vi "for_loop-2d.vi"() -> ()   [LabVIEW 2012]
panel:
  out "column  iterations":i32
  out "Rows":i32
  out "Array":i32[][](array[numeric])
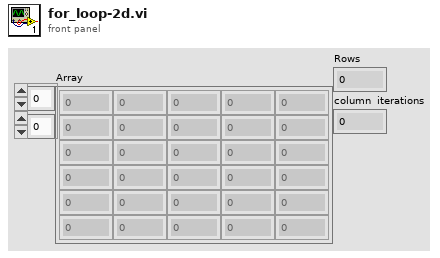
[diagram p1: front panel]
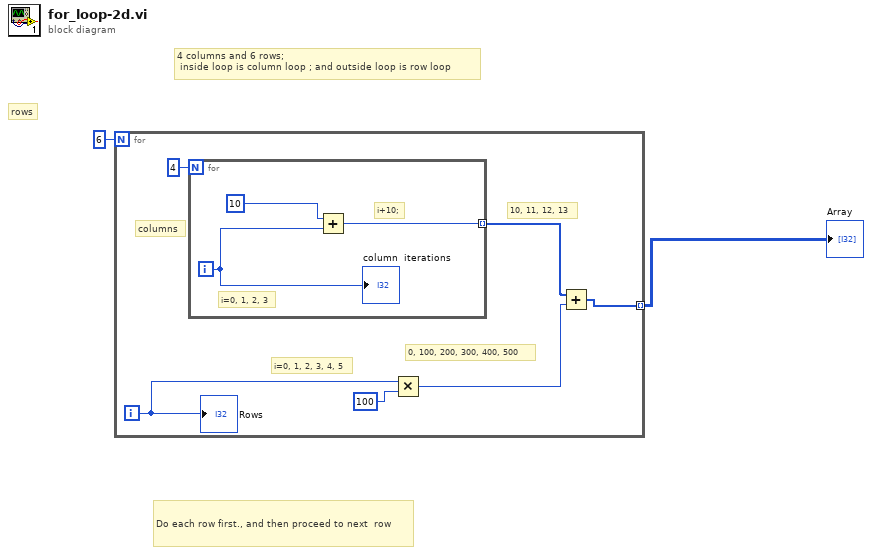
[diagram p0: block diagram]
diagram:
  # "rows"
  # "4 columns and 6 rows;\n inside loop is column loop ; and outside loop is row loop"
  # "Do each row first., and then proceed to next  row"
  n1 = for {
    N: 6 -> [_]
    tunnel: [w3] -> w1 mode=indexing
    i -> [w7]
    # "10, 11, 12, 13"
    # "0, 100, 200, 300, 400, 500"
    # "i=0, 1, 2, 3, 4, 5"
    # "columns"
    n2 = for {
      N: 4 -> [_]
      tunnel: [w9] -> w5 mode=indexing
      i -> [w11]
      # "i=0, 1, 2, 3"
      # "i+10;"
      n3 = Add(x=10, y=w11) -> (x+y=w9:i32)
      "column  iterations" <- w11
    }
    n4 = Multiply(x=w7, y=100) -> (x*y=w4:i32)
    n5 = Add(x=w5, y=w4) -> (x+y=w3:i32[])
    "Rows" <- w7
  }
  "Array" <- w1
